vi "Read GasList.vi"() -> (3 "value":T1=[{"String"="N2", "Value"=1.0}, {"String"="SF6", "Value"=0.26}, {"String"="N2O", "Value"=0.71}])   [LabVIEW 2020]
uses:
  GasList.ctl
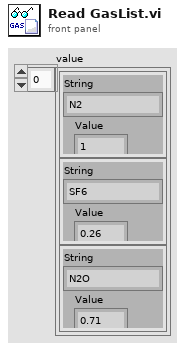
[diagram p1: front panel]
types:
  T1 = typedef "GasList.ctl" = cluster{"String":string, "Value":sgl}[]
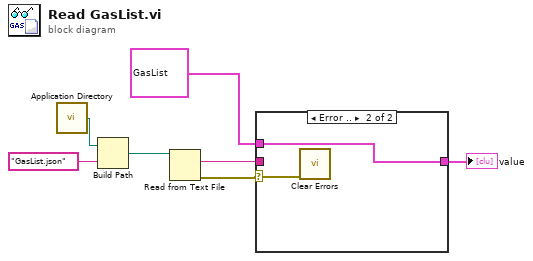
[diagram p0: block diagram]
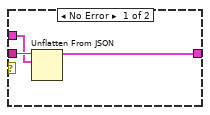
[diagram p2: hidden frame]
diagram:
  n1 = call <vilib>:"Application Directory.vi"() -> ("Application Directory"=w7:path)
  n2 = Build Path(base path=w7, name or relative path="GasList.json") -> (appended path=w5:path)
  n3 = Read from Text File(file (use dialog)=w5) -> (text=w4:string, error out=w1:errorcluster)  [unwired: 3 in, 2 out]
  n4 = case shown="Error .." w1 {
    selector: w1 -> [_ w11]
    tunnel: w4 -> [w10 _]
    tunnel: T1 [{"String"="N2", "Value"=1.0}, {"String"="SF6", "Value"=0.26}, {"String"="N2O", "Value"=0.71}] ("GasList") -> [w9 w12]
    tunnel: [w8 w12] -> w2
    frame No Error {
      n5 = Unflatten From JSON(JSON string=w10, type and defaults=w9) -> (value=w8:T1)  [unwired: 5 in, 1 out]
    }
    frame Error {
      n6 = call <vilib>:"Clear Errors.vi"("error in (no error)"=w11) -> ()  [unwired: 5 in, 2 out]
    }
  }
  "value" <- w2
